vi "CRYReport Pic Wait Frame.vi"(7 "sAction":string, 10 "vi reference":refnum<vi>) -> (1 "sData_Out":string)   [LabVIEW 2013]
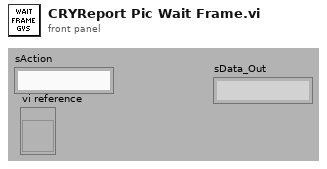
[diagram p1: front panel]
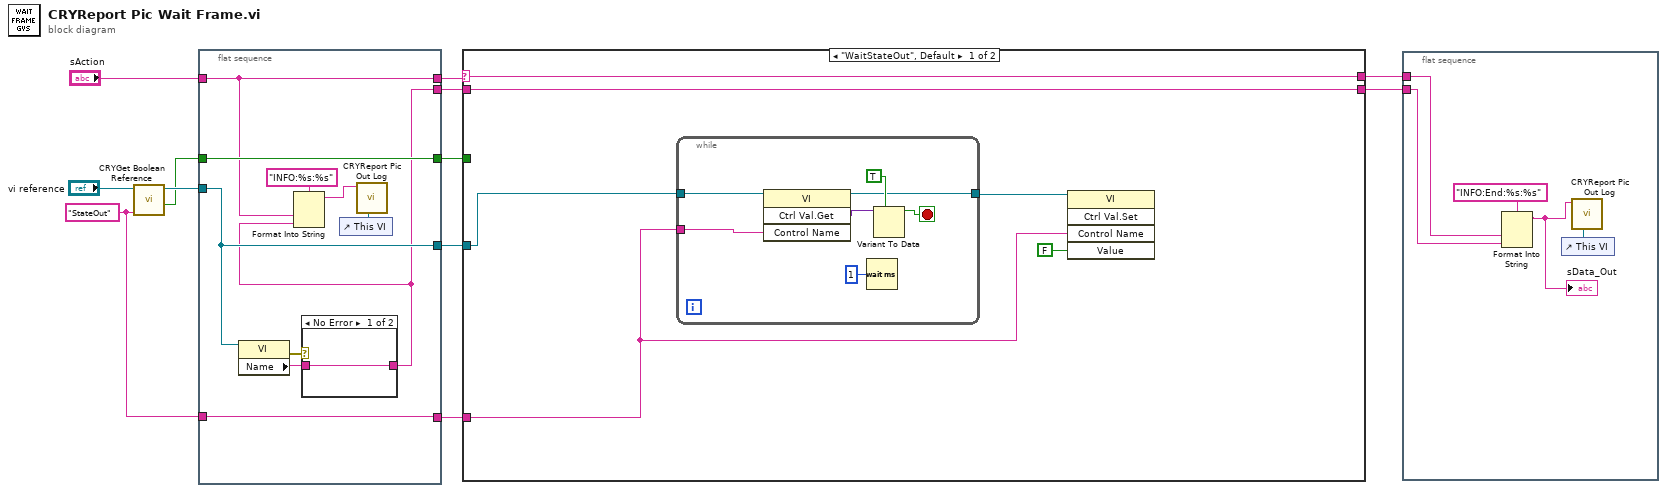
[diagram p0: block diagram]
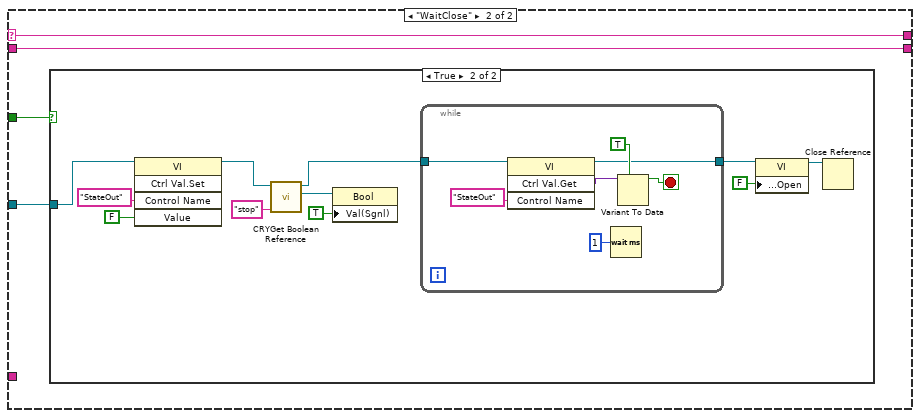
[diagram p2: hidden frame]
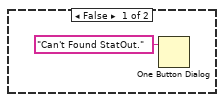
[diagram p3: hidden frame]
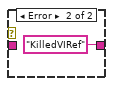
[diagram p4: hidden frame]
diagram:
  w2 = "StateOut" ("Label Name")
  n1 = call "CRYGet Boolean Reference.vi"("Label Name"=w2, "VI Refnum"="vi reference") -> ("Exist?"=w11:bool, "VI Refnum Out"=w12:refnum<vi>)  [unwired: 7 in, 1 out]
  n2 = flat-sequence {
    tunnel: [w18] -> w10
    tunnel: w12 -> [w18]
    tunnel: [w22] -> w9
    tunnel: w11 -> [w22]
    tunnel: "sAction" -> [w17]
    tunnel: [w17] -> w8
    tunnel: [w16] -> w6
    tunnel: [w13] -> w1
    tunnel: w2 -> [w13]
    frame #0 {
      n3 = property class="VI"(reference=w18) -> (error out=w20:errorcluster, "Name"=w19:string)  [unwired: 1 in, 1 out]
      n4 = case shown="No Error" w20 {
        tunnel: w19 -> [w23 _]
        tunnel: [w23 "KilledVIRef" ("sAction")] -> w16
        frame No Error {
        }
        frame Error {
        }
      }
      n5 = Format Into String(format string="INFO:%s:%s" ("string"), w17, w16) -> (resulting string=w14:string)  [unwired: 2 in, 1 out]
      n6 = control-ref of="This VI"() -> (w15:refnum<vi>)
      n7 = call "CRYReport Pic Out Log.vi"("vi reference"=w15, "sData"=w14) -> ()  [unwired: 10 in]
    }
  }
  n8 = case shown="\"WaitStateOut\", Default" w8 {
    selector: w8 -> [w30 w39]
    tunnel: w10 -> [w29 w41]
    tunnel: w9 -> [_ w40]
    tunnel: [w30 w39] -> w7
    tunnel: w6 -> [w28 w38]
    tunnel: [w28 w38] -> w5
    tunnel: w1 -> [w25 _]
    frame "WaitStateOut", Default {
      n9 = while {
        tunnel: w29 -> [w37]
        tunnel: [w32] -> w26
        tunnel: w25 -> [w31]
        stop <- w34 stop-if-true
        n10 = invoke class="VI" method="Ctrl Val.Get"(reference=w37, "Control Name"=w31) -> (reference out=w32:refnum<vi>, "Get Control Value Variant"=w36:variant)  [unwired: 2 in, 2 out]
        n11 = Wait (ms)(milliseconds to wait=u32 1) -> ()  [unwired: 1 out]
        n12 = Variant To Data(type=TRUE, Variant=w36) -> (data=w34:bool)  [unwired: 1 in, 1 out]
      }
      n13 = invoke class="VI" method="Ctrl Val.Set"(reference=w26, "Control Name"=w25, "Value"=FALSE) -> ()  [unwired: 2 in, 5 out]
    }
    frame "WaitClose" {
      n14 = case shown="True" w40 {
        tunnel: w41 -> [_ w46]
        frame False {
          n15 = One Button Dialog(message="Can't Found StatOut.") -> ()  [unwired: 1 in, 1 out]
        }
        frame True {
          n16 = invoke class="VI" method="Ctrl Val.Set"(reference=w46, "Control Name"="StateOut", "Value"=FALSE) -> (reference out=w48:refnum<vi>)  [unwired: 2 in, 4 out]
          n17 = call "CRYGet Boolean Reference.vi"("Label Name"="stop", "VI Refnum"=w48) -> ("Boolean Ref"=w51:refnum<vi>, "VI Refnum Out"=w47:refnum<vi>)  [unwired: 7 in, 1 out]
          n18 = property class="Bool"(reference=w51, "Val(Sgnl)"=TRUE) -> ()  [unwired: 1 in, 2 out]
          n19 = while {
            tunnel: w47 -> [w59]
            tunnel: [w54] -> w45
            stop <- w56 stop-if-true
            n20 = invoke class="VI" method="Ctrl Val.Get"(reference=w59, "Control Name"="StateOut") -> (reference out=w54:refnum<vi>, "Get Control Value Variant"=w58:variant)  [unwired: 2 in, 2 out]
            n21 = Wait (ms)(milliseconds to wait=u32 1) -> ()  [unwired: 1 out]
            n22 = Variant To Data(type=TRUE, Variant=w58) -> (data=w56:bool)  [unwired: 1 in, 1 out]
          }
          n23 = property class="VI"(reference=w45, "Front Panel.Open"=FALSE ("Front Panel Window:Open")) -> (reference out=w43:refnum<vi>)  [unwired: 1 in, 1 out]
          n24 = Close Reference(reference=w43) -> ()  [unwired: 1 in, 1 out]
        }
      }
    }
  }
  n25 = flat-sequence {
    tunnel: w7 -> [w64]
    tunnel: w5 -> [w63]
    frame #0 {
      n26 = Format Into String(format string="INFO:End:%s:%s" ("string"), w64, w63) -> (resulting string=w61:string)  [unwired: 2 in, 1 out]
      "sData_Out" <- w61
      n27 = control-ref of="This VI"() -> (w62:refnum<vi>)
      n28 = call "CRYReport Pic Out Log.vi"("vi reference"=w62, "sData"=w61) -> ()  [unwired: 10 in]
    }
  }
